vi "rdb_json_decode_key.vi"(8 "error in (no error)":errorcluster, 9 "offset (0)":i32, 11 "json":string) -> (0 "error out":errorcluster, 1 "offset past match":i32, 2 "key":string)   [LabVIEW 2017]
uses:
  <vilib>/Utility/error.llb/Error Cluster From Error Code.vi
  <vilib>/regexp/Match Regular Expression.xnode
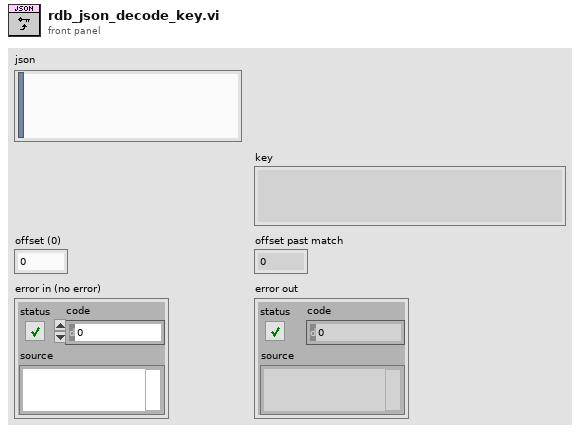
[diagram p1: front panel]
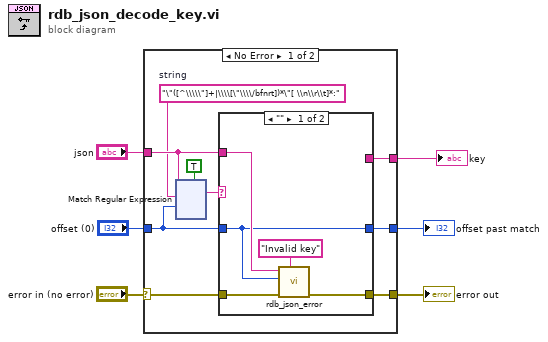
[diagram p0: block diagram]
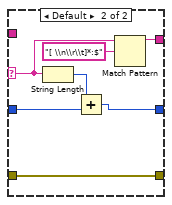
[diagram p2: hidden frame]
diagram:
  n1 = case shown="No Error" "error in (no error)" {
    selector: "error in (no error)" -> [w14 w143]
    tunnel: [w15 w143] -> w6
    tunnel: [w13 _] -> w4
    tunnel: "json" -> [w12 _]
    tunnel: "offset (0)" -> [w10 w142]
    tunnel: [w11 w142] -> w1
    frame No Error {
      w9 = "\"([^\\\\\"]+|\\\\[\"\\\\/bfnrt])*\"[ \\n\\r\\t]*:"  # string
      n2 = xnode "Match Regular Expression"("input string"=w12, "regular expression"=w9, "offset (0)"=w10, "multiline? (F)"=TRUE) -> ("whole match"=w7:string)  [unwired: 2 in, 4 out]
      n3 = case shown="\"\"" w7 {
        selector: w7 -> [_ w22]
        tunnel: w12 -> [w18 _]
        tunnel: [w19 w27] -> w15
        tunnel: w14 -> [w20 w27]
        tunnel: [_ w24] -> w13
        tunnel: w10 -> [w17 w26]
        tunnel: [w17 w25] -> w11
        frame "" {
          n4 = call "rdb_json_error.vi"("message"="Invalid key", "error in (no error)"=w20, "offset (0)"=w17, "json"=w18) -> ("error out"=w19:errorcluster)  [unwired: 7 in]
        }
        frame Default {
          n5 = String Length(string=w22) -> (length=w21:i32)
          n6 = Add(x=w21, y=w26) -> (x+y=w25:i32)
          n7 = Match Pattern(string=w22, regular expression="[ \\n\\r\\t]*:$") -> (before substring=w24:string)  [unwired: 1 in, 3 out]
        }
      }
    }
    frame Error {
    }
  }
  "error out" <- w6
  "key" <- w4
  "offset past match" <- w1
